vi "Level Color.vi"(10 "Numeric Indicator Reference":refnum<vi>, 11 "LVL Chart Refernce":refnum<vi>) -> ()   [LabVIEW 2016, in "Instrument.Oxford1820 UI.lvclass"]
uses:
  Instrument.Oxford1820 UI.lvclass
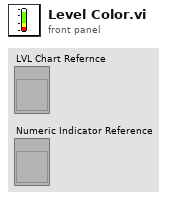
[diagram p1: front panel]
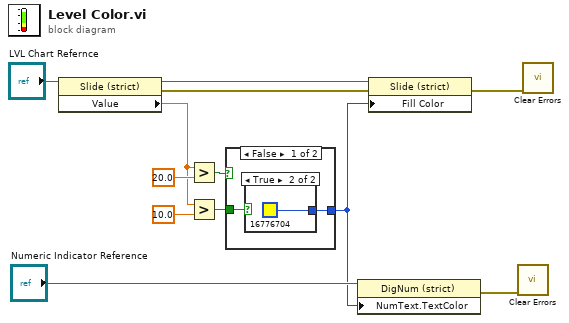
[diagram p0: block diagram]
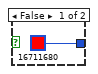
[diagram p2: hidden frame]
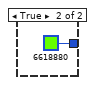
[diagram p3: hidden frame]
diagram:
  n1 = property on="Property Node" class="Slide (strict)"(reference="LVL Chart Refernce") -> (reference out=w11:refnum<vi>, error out=w4:errorcluster, "Value"=w1:dbl)  [unwired: 1 in]
  n2 = Greater?(x=w1, y=20.0) -> (0:w6:bool)
  n3 = Greater?(x=w1, y=10.0) -> (0:w5:bool)
  n4 = case shown="False" w6 {
    tunnel: [w13 u32 6618880] -> w9
    tunnel: w5 -> [w14 _]
    frame False {
      n5 = case shown="True" w14 {
        tunnel: [u32 16711680 u32 16776704] -> w13
        frame False {
        }
        frame True {
        }
      }
    }
    frame True {
    }
  }
  n6 = property on="Property Node" class="DigNum (strict)"(reference="Numeric Indicator Reference", "NumText.TextColor"=w9) -> (error out=w2:errorcluster)  [unwired: 1 in, 1 out]
  n7 = property on="Property Node" class="Slide (strict)"(reference=w11, error in=w4, "Fill Color"=w9) -> (error out=w3:errorcluster)  [unwired: 1 out]
  n8 = call <vilib>:"Clear Errors.vi"("error in (no error)"=w2) -> ()  [unwired: 5 in, 2 out]
  n9 = call <vilib>:"Clear Errors.vi"("error in (no error)"=w3) -> ()  [unwired: 5 in, 2 out]
